vi "AnzahlMfcVentile.vi"(0 "Array":string[][](array[string])) -> (1 "Anzahal Mfc's":i32, 2 "Anzahl Ventile":i32)   [LabVIEW 2017]
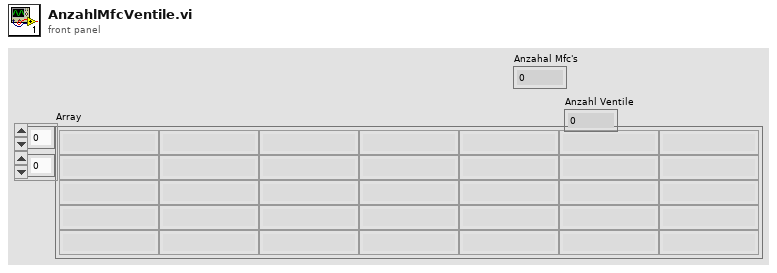
[diagram p1: front panel]
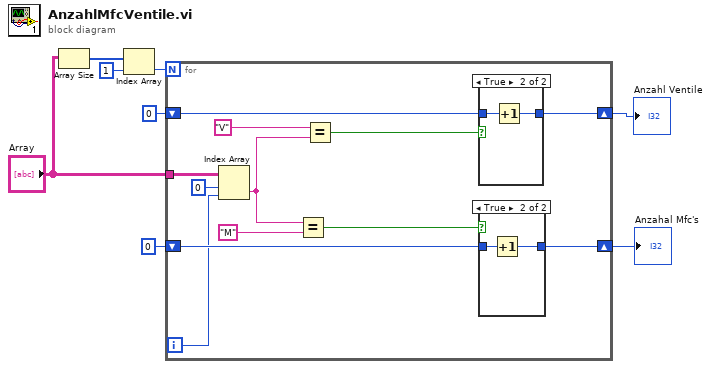
[diagram p0: block diagram]
diagram:
  n1 = Array Size(array="Array") -> (size(s)=w3:i32[])
  n2 = Index Array(array=w3, index=1) -> (element=w1:i32)
  n3 = for {
    N: w1 -> [_]
    tunnel: "Array" -> [w19]
    shift-right: [w16] -> w7
    shift-left: 0 -> [w17]
    shift-right: [w12] -> w6
    shift-left: 0 -> [w11]
    i -> [w14]
    n4 = Index Array(array=w19, index (row)=0, index (col)=w14) -> (element=w9:string)
    n5 = Equal?(x=w9, y="M") -> (x = y?=w18:bool)
    n6 = Equal?(x="V", y=w9) -> (x = y?=w13:bool)
    n7 = case shown="True" w13 {
      tunnel: w11 -> [w21 w23]
      tunnel: [w21 w22] -> w12
      frame False {
      }
      frame True {
        n8 = Increment(x=w23) -> (x+1=w22:i32)
      }
    }
    n9 = case shown="True" w18 {
      tunnel: w17 -> [w24 w26]
      tunnel: [w24 w25] -> w16
      frame False {
      }
      frame True {
        n10 = Increment(x=w26) -> (x+1=w25:i32)
      }
    }
  }
  "Anzahal Mfc's" <- w7
  "Anzahl Ventile" <- w6
